vi "HTML Report Get Wildcard Search Pattern.vi"(3 "literal string":string) -> (1 "regular expression":string)   [LabVIEW 2020, in "NI_ReportGenerationCore.lvlib"]
doc: "Builds a regular expression (used by Match Pattern) to match a literal string.\n\nWhen match case is FALSE, the regular expression will perform a case-insensitive match."
uses:
  NI_ReportGenerationCore.lvlib
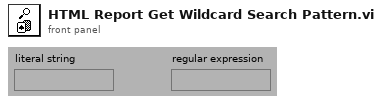
[diagram p1: front panel]
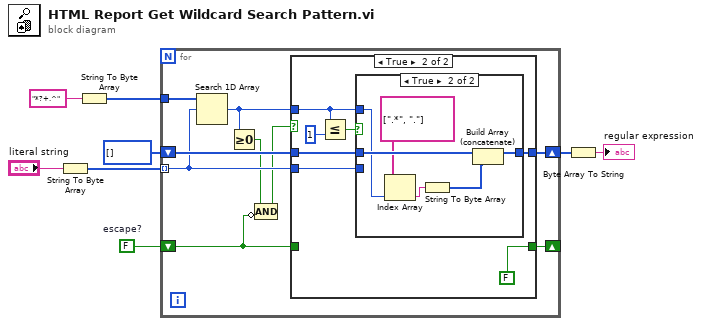
[diagram p0: block diagram]
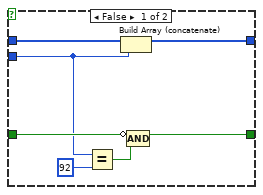
[diagram p2: hidden frame]
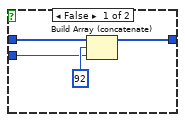
[diagram p3: hidden frame]
diagram:
  w3 = FALSE  # escape?
  n1 = String To Byte Array(string="literal string") -> (unsigned byte array=w1:u8[])
  n2 = String To Byte Array(string="*?+.^") -> (unsigned byte array=w7:u8[])
  n3 = for {
    shift-right: [w14] -> w5
    shift-left: u8[] [] -> [w16]
    tunnel: w7 -> [w17]
    tunnel: w1 -> [w15] mode=indexing
    shift-right: [w13] -> _
    shift-left: w3 -> [w12]
    n4 = Search 1D Array(1D array=w17, element=w15) -> (index of element=w9:i32)  [unwired: 1 out]
    n5 = Greater Or Equal To 0?(x=w9) -> (x >= 0?=w11:bool)
    n6 = Compound Arithmetic op=AND(w11, invert w12) -> (w10:bool)
    n7 = case shown="True" w10 {
      tunnel: w16 -> [w24 w31]
      tunnel: w15 -> [w18 w30]
      tunnel: [w23 w29] -> w14
      tunnel: w12 -> [w21 _]
      tunnel: [w19 FALSE] -> w13
      tunnel: w9 -> [_ w25]
      frame False {
        n8 = Equal?(x=w18, y=u8 92) -> (x = y?=w20:bool)
        n9 = Build Array (concatenate)(w24, w18) -> (w23:u8[])
        n10 = Compound Arithmetic op=AND(invert w21, w20) -> (w19:bool)
      }
      frame True {
        n11 = Less Or Equal?(x=w25, y=1) -> (x <= y?=w26:bool)
        n12 = case shown="True" w26 {
          tunnel: [w34 w40] -> w29
          tunnel: w30 -> [w33 _]
          tunnel: w31 -> [w32 w41]
          tunnel: w25 -> [_ w39]
          frame False {
            n13 = Build Array (concatenate)(w32, u8 92, w33) -> (w34:u8[])
          }
          frame True {
            n14 = Index Array(array=string[] [".*", "."], index=w39) -> (element=w37:string)
            n15 = String To Byte Array(string=w37) -> (unsigned byte array=w36:u8[])
            n16 = Build Array (concatenate)(w41, w36) -> (w40:u8[])
          }
        }
      }
    }
  }
  n17 = Byte Array To String(unsigned byte array=w5) -> (string=→"regular expression":string)
